vi "passifeqal - StringArray.vi"(6 "custom report message (\"\")":string, 7 "error in (no error)":errorcluster, 8 "y":string[](array[string]), 9 "x":string[](array[string]), 10 "testcase-Basic-Function in":refnum<class "testcase-Basic-Function.lvclass">) -> (0 "error out":errorcluster, 3 "testcase-Basic-Function out":refnum<class "testcase-Basic-Function.lvclass">)   [LabVIEW 2017]
uses:
  _previous/testcase-Basic-Function/testcase-Basic-Function.lvclass
  src/user.lib/_NEVSTOP/Communicable State Machine(CSM)/Communicable State Machine.lvlib
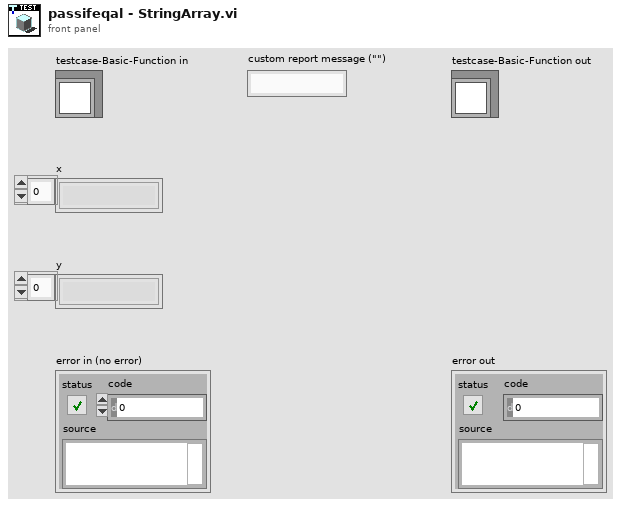
[diagram p1: front panel]
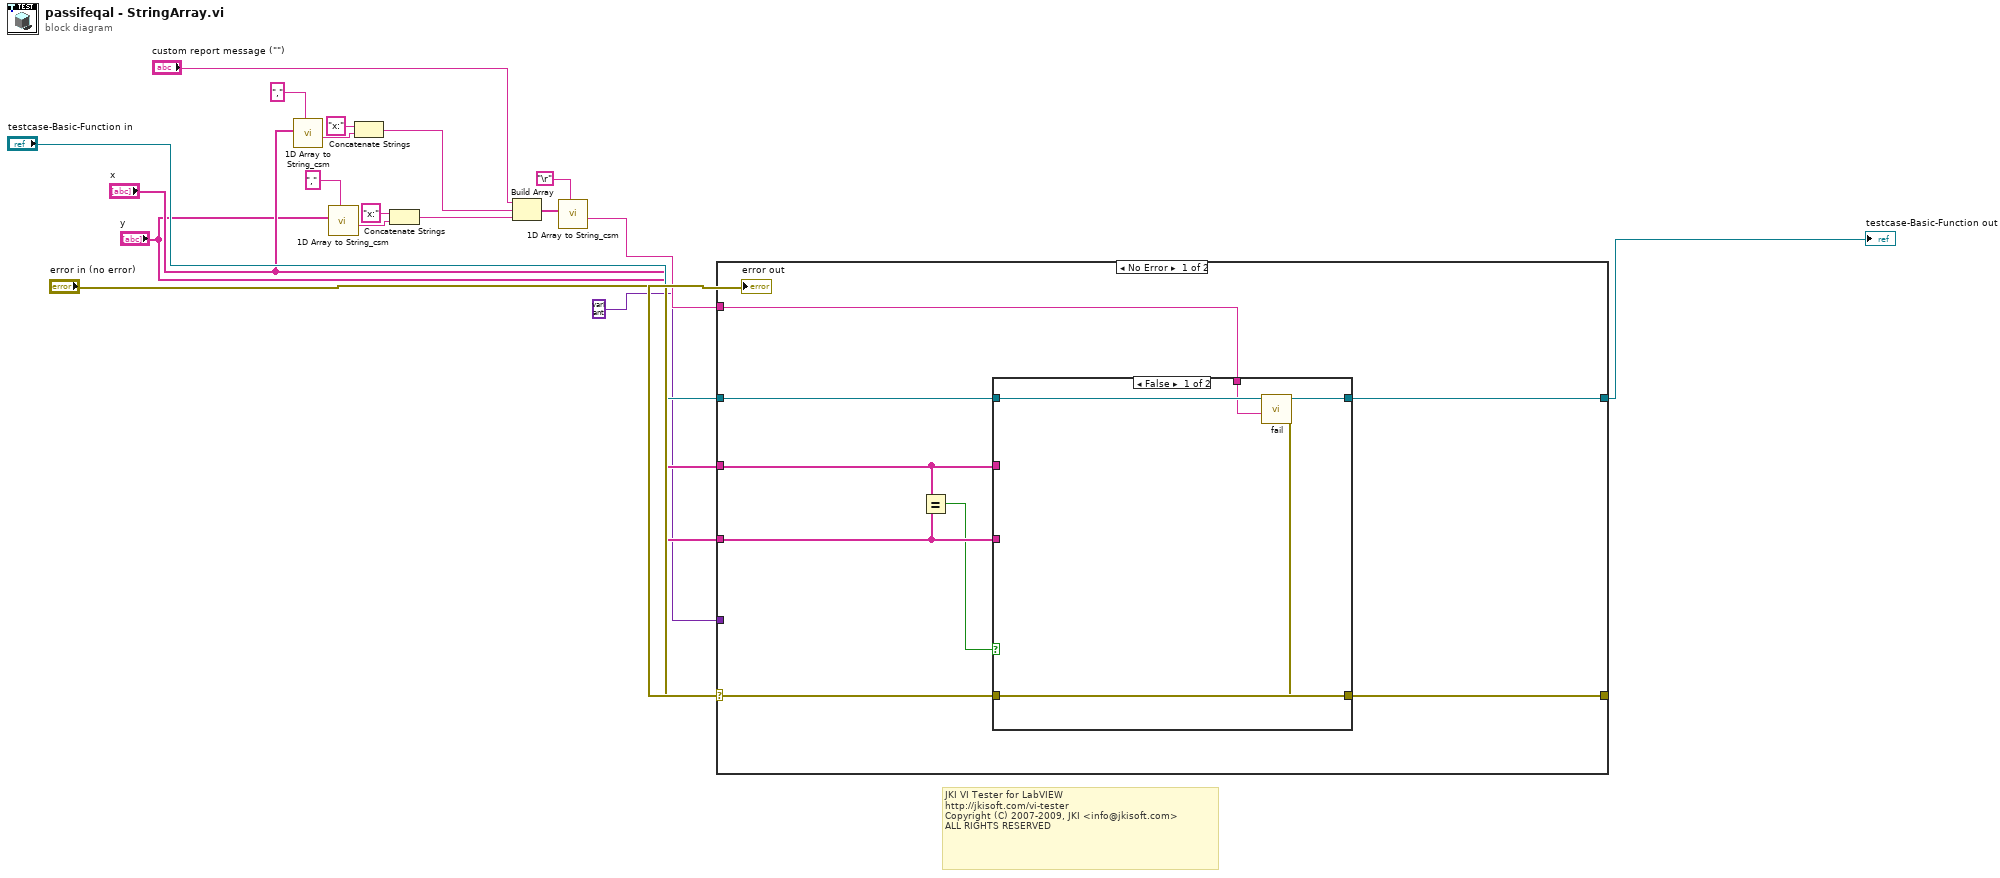
[diagram p0: block diagram]
diagram:
  # "JKI VI Tester for LabVIEW\nhttp://jkisoft.com/vi-tester\nCopyright (C) 2007-2009, JKI <info@jkisoft.com>\nALL RIGHTS RESERVED"
  n1 = call "1D Array to String_csm.vi"("delimiter (Tab)"=",", "Array of Strings"="x") -> ("delimited string"=w14:string)  [unwired: 9 in]
  n2 = call "1D Array to String_csm.vi"("delimiter (Tab)"=",", "Array of Strings"="y") -> ("delimited string"=w9:string)  [unwired: 9 in]
  n3 = Concatenate Strings("x:" ("string"), w14) -> (w6:string)
  n4 = Concatenate Strings("x:" ("string"), w9) -> (w7:string)
  n5 = Build Array("custom report message (\"\")", w6, w7) -> (w5:string[])
  n6 = call "1D Array to String_csm.vi"("delimiter (Tab)"="\r", "Array of Strings"=w5) -> ("delimited string"=w3:string)  [unwired: 9 in]
  n7 = case shown="No Error" "error in (no error)" {
    selector: "error in (no error)" -> [w25 w35]
    tunnel: [w24 w35] -> w19
    tunnel: [w22 w34] -> w18
    tunnel: "testcase-Basic-Function in" -> [w23 w34]
    tunnel: variant ("delta (optional)") -> [_ _]
    tunnel: "x" -> [w27 _]
    tunnel: "y" -> [w26 _]
    tunnel: w3 -> [w20 _]
    frame No Error {
      n8 = Equal?(x=w27, y=w26) -> (x = y?=w21:bool)
      n9 = case shown="False" w21 {
        tunnel: w25 -> [_ w32]
        tunnel: [w31 w32] -> w24
        tunnel: w23 -> [w30 w33]
        tunnel: [w29 w33] -> w22
        tunnel: w27 -> [_ _]
        tunnel: w26 -> [_ _]
        tunnel: w20 -> [w28 _]
        frame False {
          n10 = call-dynamic "fail.vi"("message (\"\")"=w28, "TestCase in"=w30) -> ("error out"=w31:errorcluster, "TestCase out"=w29:refnum<class "testcase-Basic-Function.lvclass">)  [unwired: 8 in]
        }
        frame True {
        }
      }
    }
    frame Error {
    }
  }
  "error out" <- w19
  "testcase-Basic-Function out" <- w18
